vi "Services.Settings.CreateChannelNames.vi"(7 "Diagnostic Protocol":T5, 11 "Type":T4) -> (3 "Settings Channels":T1[](array[typedef]))   [LabVIEW 2019, in "Diagnostics Addon System Explorer.lvlib"]
uses:
  Diagnostics Addon System Explorer.lvlib
  Addon Shared/Types/Protocol.ctl
  Addon Shared/Types/Type.ctl
  Addon Shared/Types/Settings.Channel.ctl
  <vilib>/NI VeriStand/Custom Device API/Custom Device Channel.ctl
  <vilib>/NI VeriStand/Custom Device API/Custom Device Channel Type.ctl
  Types/Service.Settings.ctl
  <vilib>/NI VeriStand/Custom Device API/Custom Device API.lvlib
  Addon Shared/Diagnostics Addon Shared.lvlib
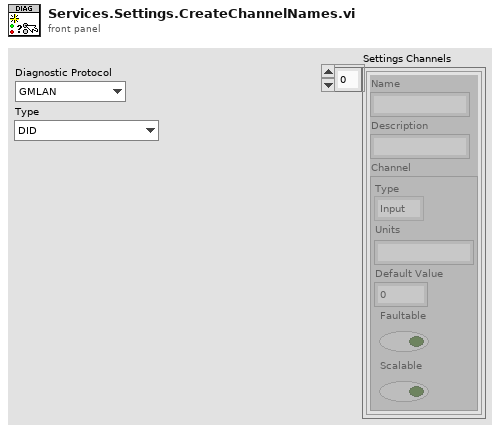
[diagram p1: front panel]
types:
  T1 = typedef "Diagnostics Addon Shared.lvlib/Settings.Channel.ctl" = cluster{"Name":string, "Description":string, "Channel":T2}
  T2 = typedef "Custom Device API.lvlib/Custom Device Channel.ctl" = cluster{"Type":T3, "Units":string, "Default Value":dbl, "Faultable":bool, "Scalable":bool}
  T3 = typedef "Custom Device API.lvlib/Custom Device Channel Type.ctl" = enum16{"Input", "Output"}
  T4 = typedef "Diagnostics Addon Shared.lvlib/Type.ctl" = enum16{"DID", "CDID", "PID", "CPID", "Read Memory", "Write Memory", "IO Control", "Routine Start", "Routine Request", "Routine Stop", "User Defined", "DTC Control", "Clear DTCs", "Read DTCs", "Start DTCs", "DTC Change Count", "Tester Present", "Unlock ECU", "Reset ECU", "Diag Session Control", "Communication Control", "DPID Control", "Poll Control", "Diag CAN Control"}
  T5 = typedef "Diagnostics Addon Shared.lvlib/Protocol.ctl" = enum16{"GMLAN", "KWP-2000", "UDS", "User-Defined"}
  T6 = typedef "Diagnostics Addon System Explorer.lvlib/Service.Settings.ctl" = cluster{"Name":string, "Default":i64, "Units":string, "Description":string}
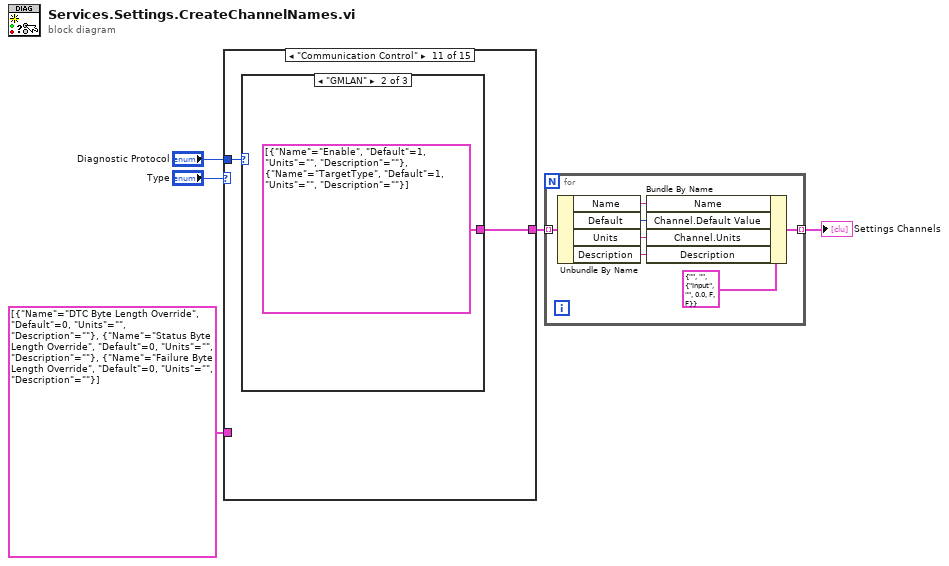
[diagram p0: block diagram]
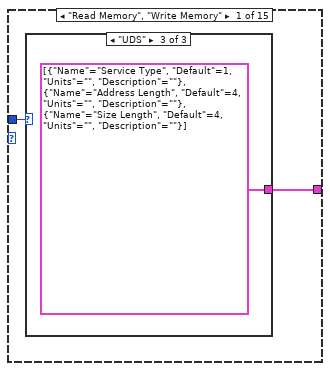
[diagram p2: hidden frame]
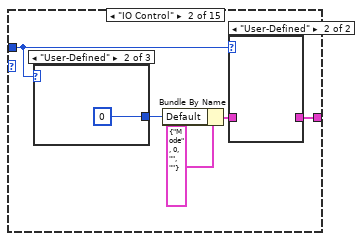
[diagram p5: hidden frame]
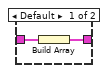
[diagram p6: hidden frame]
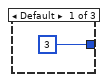
[diagram p7: hidden frame]
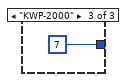
[diagram p8: hidden frame]
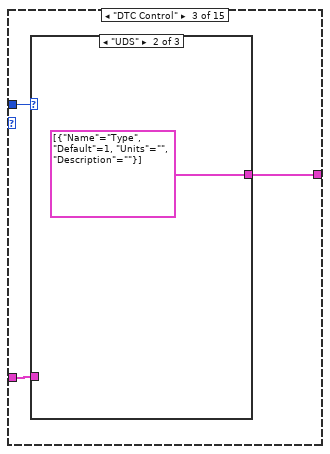
[diagram p9: hidden frame]
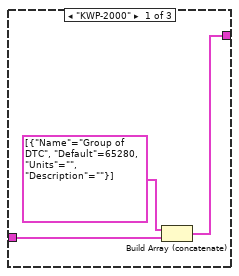
[diagram p10: hidden frame]
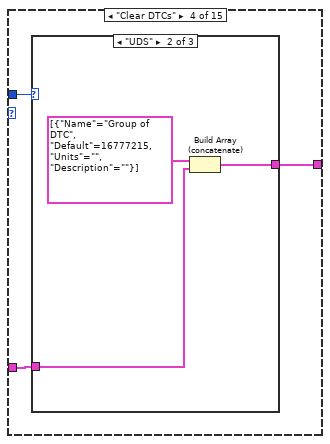
[diagram p12: hidden frame]
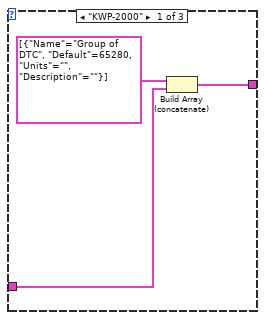
[diagram p13: hidden frame]
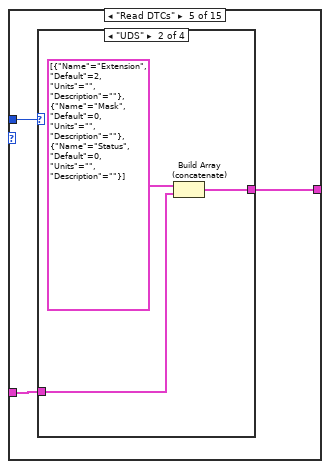
[diagram p15: hidden frame]
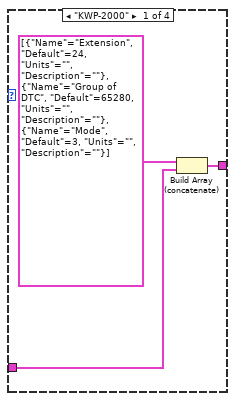
[diagram p16: hidden frame]
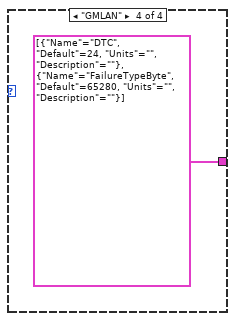
[diagram p18: hidden frame]
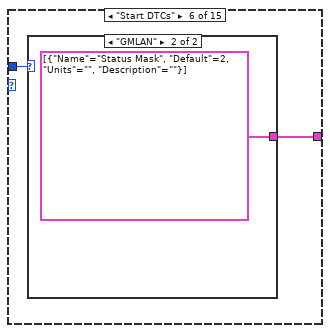
[diagram p19: hidden frame]
diagram:
  n1 = case shown="\"Communication Control\"" "Type" {
    tunnel: "Diagnostic Protocol" -> [w7 w13 w21 w28 w37 w45 w48 w51 w55 w58 w61 w65 _ _ _]
    tunnel: [w6 w9 w19 w27 w36 w46 w49 w52 w56 w59 w62 w66 T6[] [{"Name"="Enable", "Default"=0, "Units"="", "Description"=""}] T6[] [{"Name"="Enable", "Default"=1, "Units"="", "Description"=""}] _] -> w3
    tunnel: T6[] [{"Name"="DTC Byte Length Override", "Default"=0, "Units"="", "Description"=""}, {"Name"="Status Byte Length Override", "Default"=0, "Units"="", "Description"=""}, {"Name"="Failure Byte Length Override", "Default"=0, "Units"="", "Description"=""}] -> [_ _ w20 w26 w35 _ _ _ _ _ _ _ _ _ _]
    frame "Read Memory", "Write Memory" {
      n2 = case shown="\"UDS\"" w7 {
        tunnel: [_ _ T6[] [{"Name"="Service Type", "Default"=1, "Units"="", "Description"=""}, {"Name"="Address Length", "Default"=4, "Units"="", "Description"=""}, {"Name"="Size Length", "Default"=4, "Units"="", "Description"=""}]] -> w6
        frame Default {
        }
        frame "User-Defined" {
        }
        frame "UDS" {
        }
      }
    }
    frame "IO Control" {
      n3 = case shown="\"User-Defined\"" w13 {
        tunnel: [i64 3 ("Value") i64 0 ("Value") i64 7 ("Value")] -> w11
        frame Default {
        }
        frame "User-Defined" {
        }
        frame "KWP-2000" {
        }
      }
      n4 = Bundle By Name(cluster=T6 {"Name"="Mode", "Default"=0, "Units"="", "Description"=""}, "Default"=w11) -> (w10:T6)
      n5 = case shown="\"User-Defined\"" w13 {
        tunnel: w10 -> [w14 _]
        tunnel: [w15 _] -> w9
        frame Default {
          n6 = Build Array(w14) -> (w15:T6[])
        }
        frame "User-Defined" {
        }
      }
    }
    frame "DTC Control" {
      n7 = case shown="\"UDS\"" w21 {
        tunnel: [w22 T6[] [{"Name"="Type", "Default"=1, "Units"="", "Description"=""}] _] -> w19
        tunnel: w20 -> [w23 _ _]
        frame "KWP-2000" {
          n8 = Build Array (concatenate)(T6[] [{"Name"="Group of DTC", "Default"=65280, "Units"="", "Description"=""}], w23) -> (w22:T6[])
        }
        frame "UDS" {
        }
        frame "GMLAN", "User-Defined" {
        }
      }
    }
    frame "Clear DTCs" {
      n9 = case shown="\"UDS\"" w28 {
        tunnel: [w29 w32 _] -> w27
        tunnel: w26 -> [w31 w34 _]
        frame "KWP-2000" {
          n10 = Build Array (concatenate)(T6[] [{"Name"="Group of DTC", "Default"=65280, "Units"="", "Description"=""}], w31) -> (w29:T6[])
        }
        frame "UDS" {
          n11 = Build Array (concatenate)(T6[] [{"Name"="Group of DTC", "Default"=16777215, "Units"="", "Description"=""}], w34) -> (w32:T6[])
        }
        frame Default {
        }
      }
    }
    frame "Read DTCs" {
      n12 = case shown="\"UDS\"" w37 {
        tunnel: [w38 w41 _ T6[] [{"Name"="DTC", "Default"=24, "Units"="", "Description"=""}, {"Name"="FailureTypeByte", "Default"=65280, "Units"="", "Description"=""}]] -> w36
        tunnel: w35 -> [w40 w43 _ _]
        frame "KWP-2000" {
          n13 = Build Array (concatenate)(T6[] [{"Name"="Extension", "Default"=24, "Units"="", "Description"=""}, {"Name"="Group of DTC", "Default"=65280, "Units"="", "Description"=""}, {"Name"="Mode", "Default"=3, "Units"="", "Description"=""}], w40) -> (w38:T6[])
        }
        frame "UDS" {
          n14 = Build Array (concatenate)(T6[] [{"Name"="Extension", "Default"=2, "Units"="", "Description"=""}, {"Name"="Mask", "Default"=0, "Units"="", "Description"=""}, {"Name"="Status", "Default"=0, "Units"="", "Description"=""}], w43) -> (w41:T6[])
        }
        frame Default {
        }
        frame "GMLAN" {
        }
      }
    }
    frame "Start DTCs" {
      n15 = case shown="\"GMLAN\"" w45 {
        tunnel: [_ T6[] [{"Name"="Status Mask", "Default"=2, "Units"="", "Description"=""}]] -> w46
        frame Default {
        }
        frame "GMLAN" {
        }
      }
    }
    frame "DTC Change Count" {
      n16 = case shown="\"GMLAN\"" w48 {
        tunnel: [_ T6[] [{"Name"="Enable", "Default"=1, "Units"="", "Description"=""}, {"Name"="Status Mask", "Default"=2, "Units"="", "Description"=""}]] -> w49
        frame Default {
        }
        frame "GMLAN" {
        }
      }
    }
    frame "Tester Present" {
      n17 = case shown="\"GMLAN\"..\"UDS\"" w51 {
        tunnel: [T6[] [{"Name"="Enable", "Default"=1, "Units"="", "Description"=""}] T6[] [{"Name"="Enable", "Default"=0, "Units"="", "Description"=""}]] -> w52
        frame "GMLAN".."UDS" {
        }
        frame "User-Defined" {
        }
      }
    }
    frame "Reset ECU" {
      n18 = case shown="\"GMLAN\"..\"UDS\"" w55 {
        tunnel: [_ T6[] [{"Name"="Mode", "Default"=1, "Units"="", "Description"=""}]] -> w56
        frame Default {
        }
        frame "GMLAN".."UDS" {
        }
      }
    }
    frame "Diag Session Control" {
      n19 = case shown="\"GMLAN\"..\"UDS\"" w58 {
        tunnel: [_ T6[] [{"Name"="Enable", "Default"=0, "Units"="", "Description"=""}, {"Name"="Mode", "Default"=3, "Units"="", "Description"=""}]] -> w59
        frame Default {
        }
        frame "GMLAN".."UDS" {
        }
      }
    }
    frame "Communication Control" {
      n20 = case shown="\"GMLAN\"" w61 {
        tunnel: [_ T6[] [{"Name"="Enable", "Default"=1, "Units"="", "Description"=""}, {"Name"="TargetType", "Default"=1, "Units"="", "Description"=""}] T6[] [{"Name"="Enable", "Default"=1, "Units"="", "Description"=""}, {"Name"="Type", "Default"=1, "Units"="", "Description"=""}, {"Name"="Comm Type", "Default"=0, "Units"="", "Description"=""}]] -> w62
        frame Default {
        }
        frame "GMLAN" {
        }
        frame "KWP-2000", "UDS" {
        }
      }
    }
    frame "DPID Control" {
      n21 = case shown="\"GMLAN\"" w65 {
        tunnel: [_ T6[] [{"Name"="Enable", "Default"=0, "Units"="", "Description"=""}]] -> w66
        frame Default {
        }
        frame "GMLAN" {
        }
      }
    }
    frame "Poll Control" {
    }
    frame "Diag CAN Control" {
    }
    frame Default {
    }
  }
  n22 = for {
    tunnel: w3 -> [w75] mode=indexing
    tunnel: [w71] -> w2 mode=indexing
    n23 = Unbundle By Name(w75) -> ("Name"=w74:string, "Default"=w73:i64, "Units"=w72:string, "Description"=w70:string)
    n24 = Bundle By Name(cluster=T1 {"Name"="", "Description"="", "Channel"={"Type"=enum."Input", "Units"="", "Default Value"=0.0, "Faultable"=FALSE, "Scalable"=FALSE}}, "Name"=w74, "Channel.Default Value"=w73, "Channel.Units"=w72, "Description"=w70) -> (w71:T1)
  }
  "Settings Channels" <- w2
